vi "Log to Excel File by name.vi"(5 "status":bool[](array[boolean]), 6 "Sequence Context":T1, 7 "data":string[](array[string]), 8 "error in":errorcluster, 9 "StepName":string, 10 "start cell":cluster{"row":i32, "column":i32}, 11 "report file path":path) -> (0 "error out":errorcluster, 2 "next cell":cluster{"row":i32, "column":i32})   [LabVIEW 2015]
uses:
  <vilib>/addons/TestStand/_TSLegacy.llb/LabVIEW Test - Sequence Context.ctl
  <vilib>/addons/TestStand/_TSUtility.llb/TestStand - Get Property Value (String Array).vi
  <vilib>/Utility/NIReport.llb/NI_report.lvclass
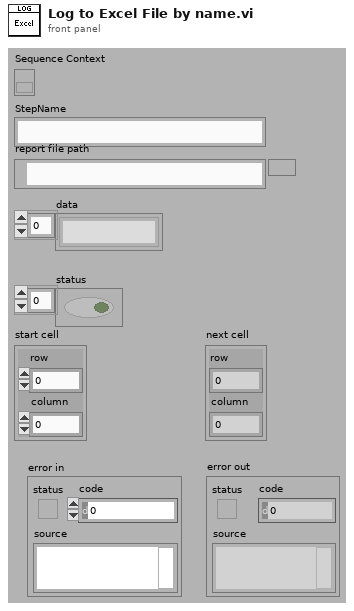
[diagram p1: front panel]
types:
  T1 = typedef "LabVIEW Test - Sequence Context.ctl" = refnum<k7>
  T2 = enum16{"Standard Report", "HTML", "Word", "Excel"}
  T3 = enum16{"maximized", "minimized", "normal", "no change"}
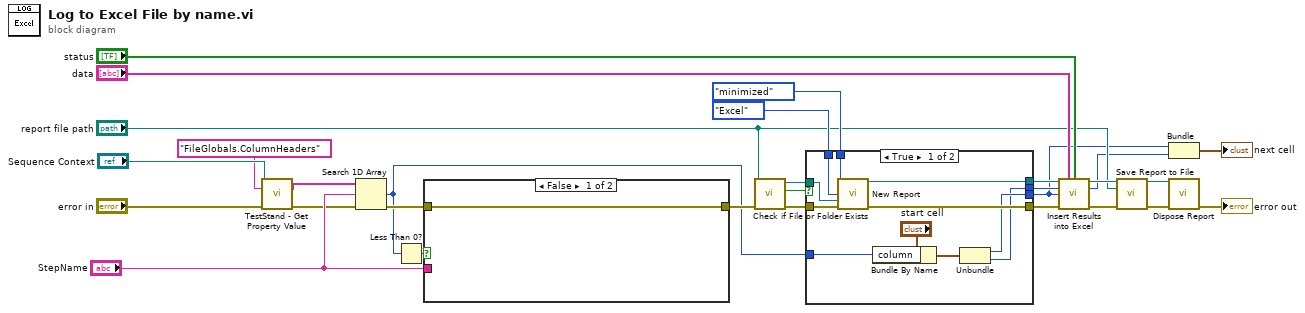
[diagram p0: block diagram]
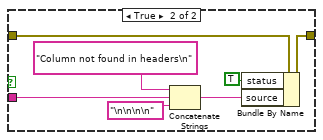
[diagram p2: hidden frame]
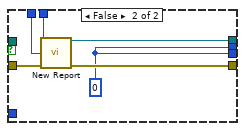
[diagram p3: hidden frame]
diagram:
  n1 = call-poly <vilib>:"TestStand - Get Property Value.vi"("Sequence Context In"="Sequence Context", "Lookup String"="FileGlobals.ColumnHeaders", "error in (no error)"="error in") -> ("Value"=w2:string[], "error out"=w5:errorcluster)  [unwired: 10 in, 1 out]
  n2 = Search 1D Array(1D array=w2, element="StepName") -> (index of element=w3:i32)  [unwired: 1 in]
  n3 = Less Than 0?(x=w3) -> (x < 0?=w1:bool)
  n4 = case shown="False" w1 {
    tunnel: w5 -> [w29 w35]
    tunnel: [w29 w36] -> w4
    tunnel: "StepName" -> [_ w33]
    frame False {
    }
    frame True {
      n5 = Concatenate Strings("Column not found in headers\n" ("string"), w33, "\n\n\n\n" ("string")) -> (w32:string)
      n6 = Bundle By Name(cluster=w35, "status"=TRUE, "source"=w32) -> (w36:errorcluster)
    }
  }
  n7 = call <vilib>:"Check if File or Folder Exists.vi"("error in (no error)"=w4, "path"="report file path") -> ("error out"=w17:errorcluster, "file or folder exists?"=w16:bool, "dup path"=w18:path)  [unwired: 7 in]
  n8 = case shown="True" w16 {
    tunnel: [w47 w53] -> w13
    tunnel: [w46 w52] -> w14
    tunnel: T3."minimized" ("window state (normal)") -> [w45 w51]
    tunnel: T2."Excel" ("report type") -> [w44 w50]
    tunnel: w18 -> [w43 _]
    tunnel: w17 -> [w42 w49]
    tunnel: [w40 w48] -> w15
    tunnel: [w41 w48] -> w12
    tunnel: w3 -> [w37 _]
    frame True {
      n9 = call <vilib>:"New Report.vi"("window state (normal)"=w45, "report type"=w44, "template (empty)"=w43, "error in (no error)"=w42) -> ("report out"=w46:refnum<class "NI_report.lvclass">, "error out"=w47:errorcluster)  [unwired: 10 in]
      n10 = Bundle By Name(cluster="start cell", "column"=w37) -> (w38:cluster{"row":i32, "column":i32})
      n11 = Unbundle(w38) -> ("row"=w41:i32, "column"=w40:i32)
    }
    frame False {
      w48 = 0 ("column")
      n12 = call <vilib>:"New Report.vi"("window state (normal)"=w51, "report type"=w50, "error in (no error)"=w49) -> ("report out"=w52:refnum<class "NI_report.lvclass">, "error out"=w53:errorcluster)  [unwired: 11 in]
    }
  }
  n13 = call "Insert Results into Excel.vi"("report in"=w14, "strings"="data", "Pass/Fail"="status", "column"=w15, "row"=w12, "error in"=w13) -> ("report out"=w27:refnum<class "NI_report.lvclass">, "column out"=w11:i32, "error out"=w28:errorcluster)  [unwired: 7 in]
  n14 = call-dynamic "Save Report to File.vi"("report in"=w27, "report file path"="report file path", "error in (no error)"=w28) -> ("report out"=w22:refnum<class "NI_report.lvclass">, "error out"=w21:errorcluster)  [unwired: 11 in]
  n15 = Bundle("column"=w12, "column out"=w11) -> (→"next cell":cluster{"column":i32, "column out":i32})  [unwired: 1 in]
  n16 = call-dynamic "Dispose Report.vi"("report in"=w22, "error in (no error)"=w21) -> ("error out"=→"error out":errorcluster)  [unwired: 13 in]
